vi "Choose date time.vi"(8 "Error In":errorcluster, 11 "Time":timestamp) -> (0 "Error Out":errorcluster, 3 "ics format Date/Time":string)   [LabVIEW 2016]
doc: "Choose date time VI converts input values to ics format string."
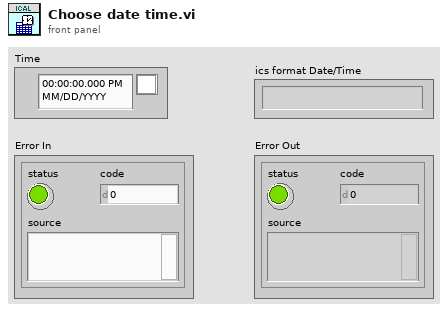
[diagram p1: front panel]
types:
  T1 = typedef "LVDateTimeRec.ctl" = cluster{"fractional second":dbl, "second":i32, "minute":i32, "hour":i32, "day of month":i32, "month":i32, "year":i32, "day of week":i32, "day of year":i32, "DST":i32}
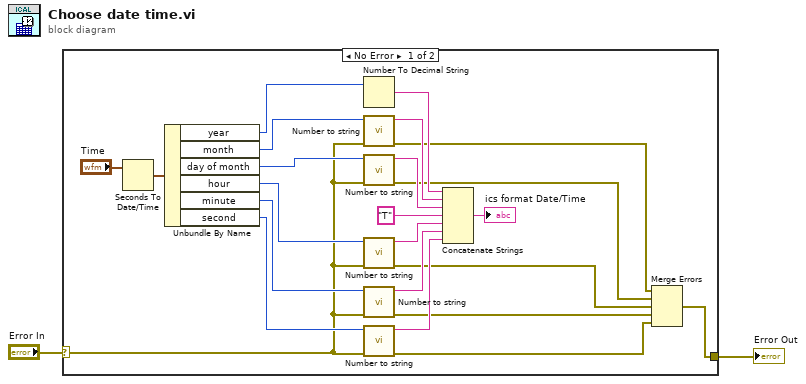
[diagram p0: block diagram]
diagram:
  n1 = case shown="No Error" "Error In" {
    selector: "Error In" -> [w9 w26]
    tunnel: [w3 w26] -> w1
    frame No Error {
      n2 = Seconds To Date/Time(time stamp (now)="Time") -> (date time rec=w21:T1)  [unwired: 1 in]
      n3 = Unbundle By Name(w21) -> ("year"=w20:i32, "month"=w19:i32, "day of month"=w18:i32, "hour"=w16:i32, "minute"=w15:i32, "second"=w17:i32)
      n4 = Number To Decimal String(number=w20) -> (decimal integer string=w22:string)  [unwired: 1 in]
      n5 = call "Number to string.vi"("Error In"=w9, "Integer"=w19) -> ("Error Out"=w8:errorcluster, "String"=w14:string)  [unwired: 8 in]
      n6 = call "Number to string.vi"("Error In"=w9, "Integer"=w18) -> ("Error Out"=w7:errorcluster, "String"=w13:string)  [unwired: 8 in]
      n7 = call "Number to string.vi"("Error In"=w9, "Integer"=w16) -> ("Error Out"=w6:errorcluster, "String"=w10:string)  [unwired: 8 in]
      n8 = call "Number to string.vi"("Error In"=w9, "Integer"=w15) -> ("Error Out"=w5:errorcluster, "String"=w11:string)  [unwired: 8 in]
      n9 = call "Number to string.vi"("Error In"=w9, "Integer"=w17) -> ("Error Out"=w4:errorcluster, "String"=w12:string)  [unwired: 8 in]
      n10 = Concatenate Strings(w22, w14, w13, "T" ("string"), w10, w11, w12) -> (→"ics format Date/Time":string)
      n11 = Merge Errors(w8, w7, w6, w5, w4) -> (w3:errorcluster)
    }
    frame Error {
    }
  }
  "Error Out" <- w1
